vi "Modified Sinc Filter (single).vi"(6 "Side Points Unit (points)":enum16{"Points", "Data"}(ring), 8 "error in (no error)":errorcluster, 10 "side points":dbl, 11 "XY-data":cluster{"X-array":dbl[], "Y-array":dbl[]}) -> (0 "error out":errorcluster, 3 "XY-data out":cluster{"X-array":dbl[], "Y-array":dbl[]} {"Y-array" format="%.2p"; "X-array" format="%.2p"})   [LabVIEW 2019, in "xy_utilities.lvlib"]
doc: "Filter <b>XY-data</b>'s Y-Array with a Savitsky-Golay FIR smoothing filter.\n\n<b>side points</b> specifies the number of data points to each side of the current data point to use for the least squares minimization. side points*2 + 1 is the length of the moving window, which must be greater than the polynomial order.\n\nWire data to the data input to determine the polymorphic instance to use or manually select the instance."
uses:
  xy_utilities.lvlib
  <vilib>/Analysis/NI_AALBase.lvlib
  <vilib>/Analysis/3filter.llb/Zero Phase Filter (DBL).vi
  <vilib>/Analysis/baseanly.llb/A x Vector.vi
  <vilib>/Analysis/baseanly.llb/Real Dot Product.vi
panel:
  in  "side points 2":i32(slide)=12 scale=0.0..50.0
  in  "polynomial order":i32(slide)=8 scale=0.0..20.0
  in  "samples":i32=300
  out "Graph":dbl[][](graph)
  in  "Stop":bool
  in  "seed":i32=-1
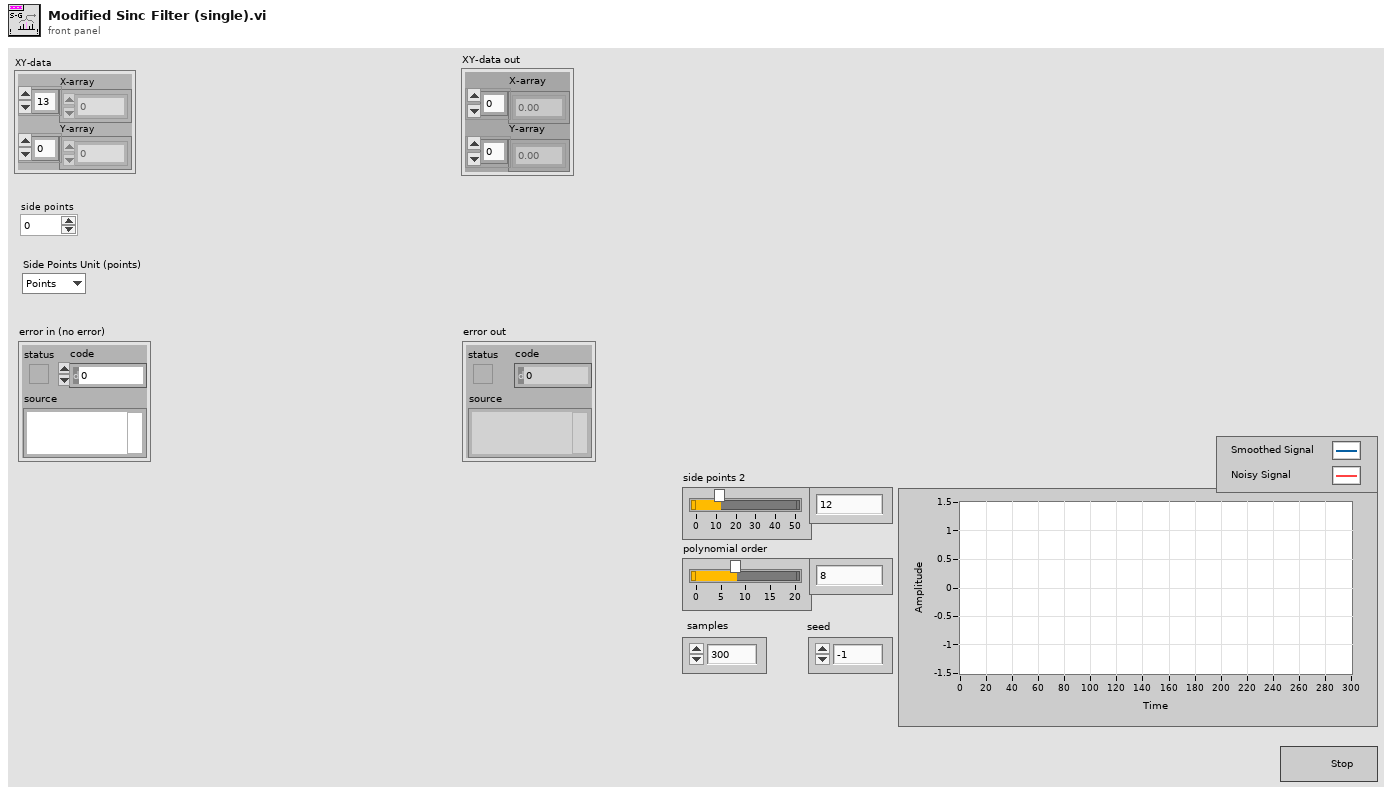
[diagram p1: front panel]
types:
  T1 = typedef "NI_Matrix.lvlib/RealMatrix.ctl" = dbl[][]
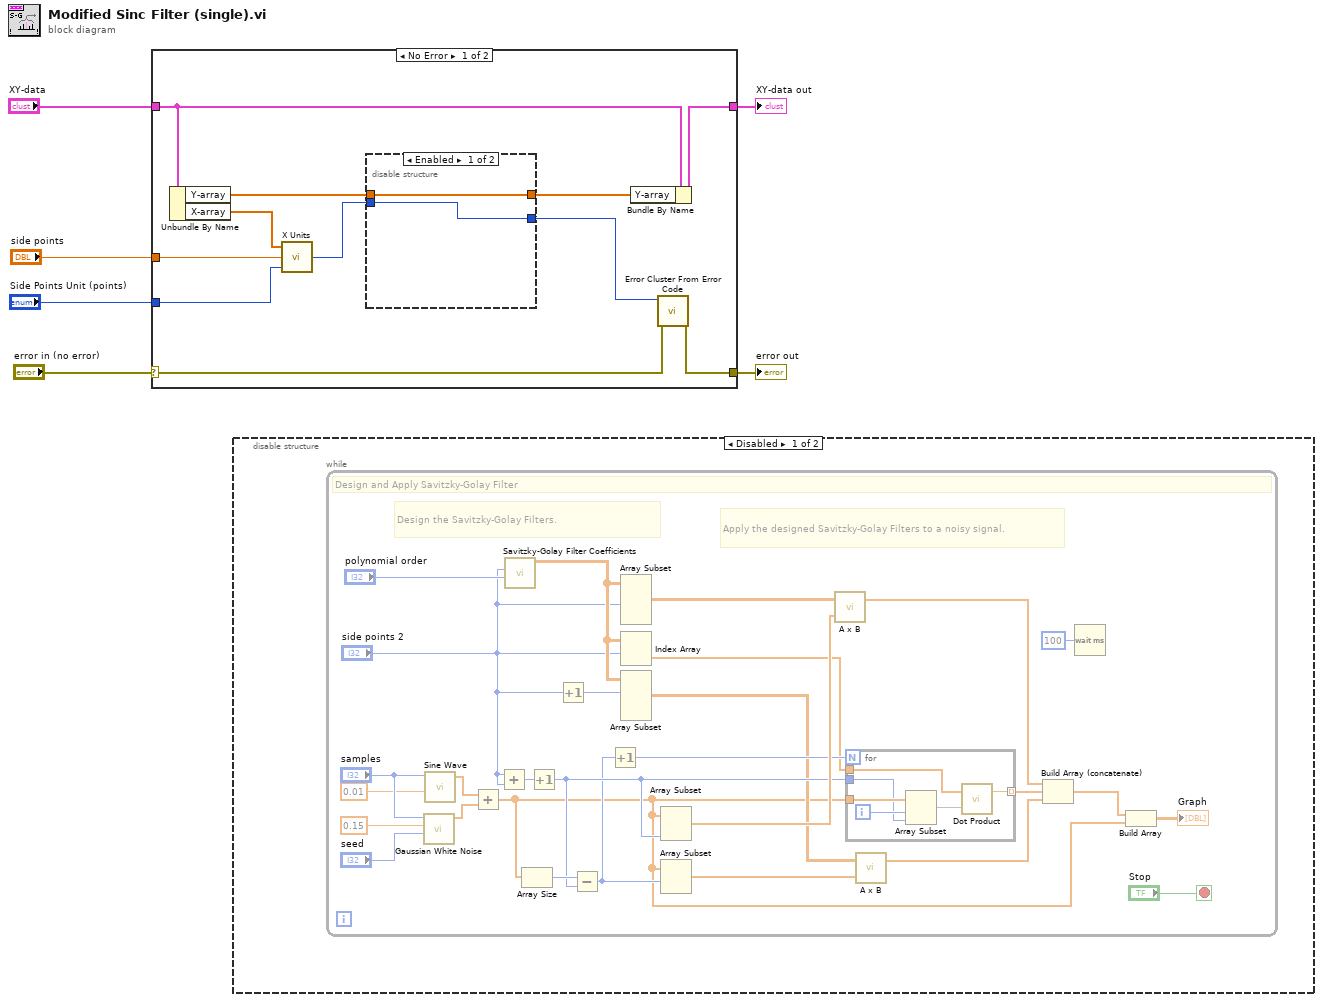
[diagram p0: block diagram]
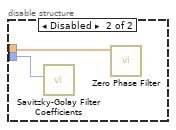
[diagram p3: hidden frame]
diagram:
  n1 = case shown="No Error" "error in (no error)" {
    selector: "error in (no error)" -> [w12 w23]
    tunnel: [w11 w23] -> w5
    tunnel: "XY-data" -> [w16 w22]
    tunnel: [w17 w22] -> w3
    tunnel: "side points" -> [w9 _]
    tunnel: "Side Points Unit (points)" -> [w7 _]
    frame No Error {
      n2 = Unbundle By Name(w16) -> ("Y-array"=w15:dbl[], "X-array"=w10:dbl[])
      n3 = call "X Units.vi"("Interval Units (points)"=w7, "Interval (h)"=w9, "X-array"=w10) -> ("h (points)"=w8:i32)
      n4 = disable-structure shown="Enabled" {
        disable-tunnel: w15 -> [w19 w21]
        disable-tunnel: [w19 _] -> w14
        disable-tunnel: [w18 _] -> w13
        disable-tunnel: w8 -> [w18 w20]
        frame Enabled {
        }
        frame Disabled {
          n5 = call <vilib>:"Savitzky-Golay Filter Coefficients.vi"("side points"=w20) -> ()  [unwired: 8 in, 3 out]
          n6 = call-poly <vilib>:"Zero Phase Filter.vi"("X"=w21) -> ()  [unwired: 9 in, 2 out]
        }
      }
      n7 = Bundle By Name(cluster=w16, "Y-array"=w14) -> (w17:cluster{"X-array":dbl[], "Y-array":dbl[]})
      n8 = call <vilib>:"Error Cluster From Error Code.vi"("error in (no error)"=w12, "error code (0)"=w13) -> ("error out"=w11:errorcluster)  [unwired: 7 in]
    }
    frame Error {
    }
  }
  "error out" <- w5
  "XY-data out" <- w3
  n9 = disable-structure shown="Disabled" {
    frame Disabled {
      n10 = while {
        stop <- "Stop" stop-if-true
        # "Apply the designed Savitzky-Golay Filters to a noisy signal."
        # "Design the Savitzky-Golay Filters."
        # "Design and Apply Savitzky-Golay Filter"
        n11 = call <vilib>:"Gaussian White Noise.vi"("seed"="seed", "standard deviation"=0.15, "samples"="samples") -> ("Gaussian noise pattern"=w33:dbl[])  [unwired: 7 in, 1 out]
        n12 = call <vilib>:"Sine Wave.vi"("samples"="samples", "frequency"=0.01 ("f")) -> ("sine wave"=w34:dbl[])  [unwired: 3 in, 2 out]
        n13 = Add(x=w34, y=w33) -> (x+y=w24:dbl[])
        n14 = Add(x="side points 2", y="side points 2") -> (x+y=w49:i32)
        n15 = call <vilib>:"Savitzky-Golay Filter Coefficients.vi"("polynomial order"="polynomial order", "side points"="side points 2") -> ("Savitzky-Golay Filters"=w42:T1)  [unwired: 7 in, 2 out]
        n16 = Array Size(array=w24) -> (size(s)=w47:i32)
        n17 = Increment(x=w49) -> (x+1=w46:i32)
        n18 = Increment(x="side points 2") -> (x+1=w50:i32)
        n19 = Subtract(x=w47, y=w46) -> (x-y=w45:i32)
        n20 = Increment(x=w45) -> (x+1=w44:i32)
        n21 = Array Subset(array=w42, length (row)="side points 2") -> (w51:T1)  [unwired: 3 in]
        n22 = Index Array(array=w42, index (row)="side points 2") -> (element=w43:dbl[])  [unwired: 1 in]
        n23 = Array Subset(array=w42, index (row)=w50) -> (w41:T1)  [unwired: 3 in]
        n24 = Array Subset(array=w24, length=w46) -> (w48:dbl[])  [unwired: 1 in]
        n25 = Array Subset(array=w24, index=w45) -> (w40:dbl[])  [unwired: 1 in]
        n26 = call-poly <vilib>:"A x B.vi"("Vector"=w48, "A"=w51) -> ("A x Vector"=w39:dbl[])  [unwired: 1 out]
        n27 = for {
          N: w44 -> [_]
          tunnel: w24 -> [w57]
          tunnel: w46 -> [w55]
          tunnel: w43 -> [w54]
          tunnel: [w52] -> w38 mode=indexing
          i -> [w56]
          n28 = Array Subset(array=w57, index=w56, length=w55) -> (w53:dbl[])
          n29 = call-poly <vilib>:"Dot Product.vi"("Y Vector"=w53, "X Vector"=w54) -> ("X * Y"=w52:dbl)  [unwired: 1 out]
        }
        n30 = call-poly <vilib>:"A x B.vi"("Vector"=w40, "A"=w41) -> ("A x Vector"=w37:dbl[])  [unwired: 1 out]
        n31 = Build Array (concatenate)(w39, w38, w37) -> (w32:dbl[])
        n32 = Wait (ms)(milliseconds to wait=u32 100) -> ()  [unwired: 1 out]
        n33 = Build Array(w32, w24) -> (→"Graph":dbl[][])
      }
    }
    frame Enabled {
    }
  }
